vi "Convert to Step Object.vi"(8 "error in":errorcluster, 10 "Step":string, 11 "Value":string) -> (0 "error out":errorcluster, 3 "STEP out":refnum<class "STEP.lvclass">)   [LabVIEW 2015]
uses:
  Reusable/Sequence/STEPS/STEP.lvclass
  Calibration/O3 Generator State/Change O3 Generator State.lvclass
  Calibration/Change Filter State/Change Filter Position.lvclass
  Calibration/Change O2 Valve.lvclass
  Calibration/Wait/Wait.lvclass
  Calibration/Wait/Wait.lvclass/Wait.ctl
  Calibration/Set QO2 Rel Flow/Set Rel QO2 flow.lvclass
  Reusable/Sequence/STEPS/LEAVES/Double/Switch DBL.lvclass/Switch DBL.ctl
  Calibration/O3 Add Valve/Ozone Addition Valve.lvclass
  Calibration/Change Spk Pos/Change Speaker Position.lvclass
  Calibration/Wait/Write Wait Time.vi
  Reusable/Sequence/STEPS/LEAVES/Double/Write val.vi
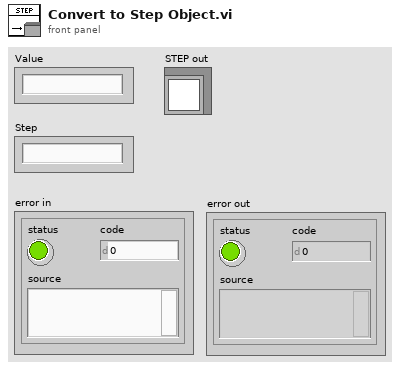
[diagram p1: front panel]
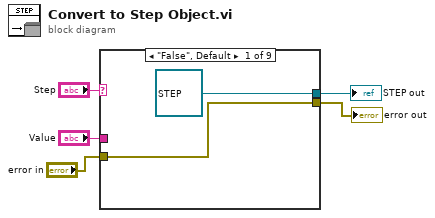
[diagram p0: block diagram]
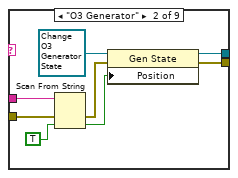
[diagram p2: hidden frame]
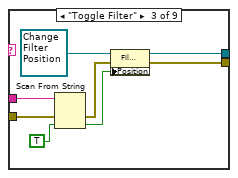
[diagram p3: hidden frame]
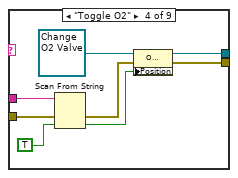
[diagram p4: hidden frame]
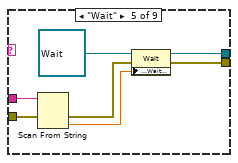
[diagram p5: hidden frame]
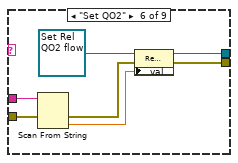
[diagram p6: hidden frame]
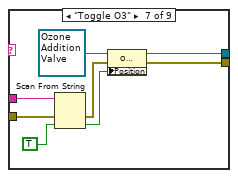
[diagram p7: hidden frame]
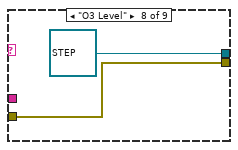
[diagram p8: hidden frame]
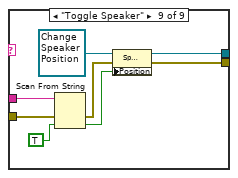
[diagram p9: hidden frame]
diagram:
  n1 = case shown="\"False\", Default" "Step" {
    tunnel: "Value" -> [_ w15 w22 w29 w37 w44 w51 _ w62]
    tunnel: [refnum<class "STEP.lvclass"> refnum ("Sequence Composition:STEP.lvclass") w11 w19 w27 w35 w42 w49 refnum<class "STEP.lvclass"> refnum ("Sequence Composition:STEP.lvclass") w59] -> w3
    tunnel: [w6 w9 w18 w26 w33 w39 w47 w54 w56] -> w2
    tunnel: "error in" -> [w6 w8 w16 w24 w32 w40 w46 w54 w58]
    frame "False", Default {
    }
    frame "O3 Generator" {
      n2 = Scan From String(input string=w15, error in=w8, default 1=TRUE) -> (error out=w10:errorcluster, output 1=w13:bool)  [unwired: 2 in, 2 out]
      n3 = property class="Gen State"(reference=refnum<class "Change O3 Generator State.lvclass"> refnum ("Gen State"), error in=w10, "Position"=w13) -> (reference out=w11:refnum<class "Change O3 Generator State.lvclass">, error out=w9:errorcluster)
    }
    frame "Toggle Filter" {
      n4 = Scan From String(input string=w22, error in=w16, default 1=TRUE) -> (error out=w17:errorcluster, output 1=w21:bool)  [unwired: 2 in, 2 out]
      n5 = property class="Filter Position"(reference=refnum<class "Change Filter Position.lvclass"> refnum ("Filter Position"), error in=w17, "Position"=w21) -> (reference out=w19:refnum<class "Change Filter Position.lvclass">, error out=w18:errorcluster)
    }
    frame "Toggle O2" {
      n6 = Scan From String(input string=w29, error in=w24, default 1=TRUE) -> (error out=w25:errorcluster, output 1=w30:bool)  [unwired: 2 in, 2 out]
      n7 = property class="O2 Valve"(reference=refnum<class "Change O2 Valve.lvclass"> refnum ("O2 Valve"), error in=w25, "Position"=w30) -> (reference out=w27:refnum<class "Change O2 Valve.lvclass">, error out=w26:errorcluster)
    }
    frame "Wait" {
      n8 = Scan From String(input string=w37, error in=w32) -> (error out=w34:errorcluster, output 1=w36:dbl)  [unwired: 3 in, 2 out]
      n9 = property class="Wait"(reference=refnum<class "Wait.lvclass"> refnum ("Wait"), error in=w34, "Data Access:Wait Time"=w36) -> (reference out=w35:refnum<class "Wait.lvclass">, error out=w33:errorcluster)
    }
    frame "Set QO2" {
      n10 = Scan From String(input string=w44, error in=w40) -> (error out=w41:errorcluster, output 1=w45:dbl)  [unwired: 3 in, 2 out]
      n11 = property class="Rel O2 Flow"(reference=refnum<class "Set Rel QO2 flow.lvclass"> refnum ("Rel O2 Flow"), error in=w41, "val"=w45) -> (reference out=w42:refnum<class "Set Rel QO2 flow.lvclass">, error out=w39:errorcluster)
    }
    frame "Toggle O3" {
      n12 = Scan From String(input string=w51, error in=w46, default 1=TRUE) -> (error out=w48:errorcluster, output 1=w52:bool)  [unwired: 2 in, 2 out]
      n13 = property class="O3 Add"(reference=refnum<class "Ozone Addition Valve.lvclass"> refnum ("O3 Add"), error in=w48, "Position"=w52) -> (reference out=w49:refnum<class "Ozone Addition Valve.lvclass">, error out=w47:errorcluster)
    }
    frame "O3 Level" {
    }
    frame "Toggle Speaker" {
      n14 = Scan From String(input string=w62, error in=w58, default 1=TRUE) -> (error out=w57:errorcluster, output 1=w60:bool)  [unwired: 2 in, 2 out]
      n15 = property class="Spk Pos"(reference=refnum<class "Change Speaker Position.lvclass"> refnum ("Spk Pos"), error in=w57, "Position"=w60) -> (reference out=w59:refnum<class "Change Speaker Position.lvclass">, error out=w56:errorcluster)
    }
  }
  "STEP out" <- w3
  "error out" <- w2
